vi "Edit Line.vi"(8 "error in":errorcluster, 10 "Line Name":string, 11 "References":T1) -> (0 "error out":errorcluster, 2 "change?":bool)   [LabVIEW 2014, in "Missing Plugin editor node.lvclass"]
doc: "This VI edits the properties of a line. It will unlink channels and tags and create new links to channels and tags."
uses:
  Missing Plugin editor node.lvclass
  <vilib>/NI/DCAF/Tag Editor Core/Table API/Table Manager/object ref.ctl
  <vilib>/NI/DCAF/Tag Editor Core/Configuration Editor/Classes/Engine Parent/Engine Parent Editor Node.lvclass
  <vilib>/NI/DCAF/Tag Editor Core/Configuration Editor/Classes/Module editor node/module editor node.lvclass
  module/configuration/Missing Plugin configuration.lvclass
  module/configuration/Missing Plugin configuration.lvclass/Missing Plugin configuration.ctl
  <vilib>/NI/Configuration Framework/serializable configuration/NISE_CEF_serializable configuration.lvclass/NISE_CEF_serializable configuration.ctl
  <vilib>/Utility/LVClass/Get LV Class Name.vi
  <vilib>/NI/Configuration Framework/error generator/NISE_error generator.vi
  <vilib>/NI/Tag Bus Module Framework/channel/TBM channel.lvclass
  <vilib>/NI/Configuration Framework/serializable configuration/NISE_CEF_serializable configuration.lvclass
  <vilib>/NI/DCAF/Tag Editor Core/Table API/Table Manager/Table Manager.lvclass
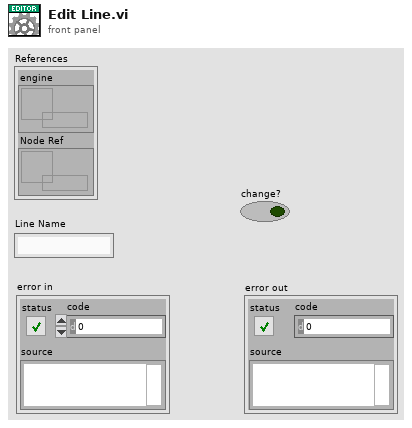
[diagram p1: front panel]
types:
  T1 = typedef "Table Manager.lvlib/Table Manager.lvclass/object ref.ctl" = cluster{"engine":refnum<data-value>, "Node Ref":refnum<data-value>}
  T2 = typedef "Missing Plugin configuration.lvclass/Line.ctl" = cluster{"channel":refnum<class "TBM channel.lvclass">}
  T3 = typedef "Missing Plugin editor node.lvclass/Mappings.ctl" = cluster{"Line":T2, "Maps":T4[]}
  T4 = typedef "Missing Plugin editor node.lvclass/Map.ctl" = cluster{"channel":refnum<class "TBM channel.lvclass">, "tag name":string}
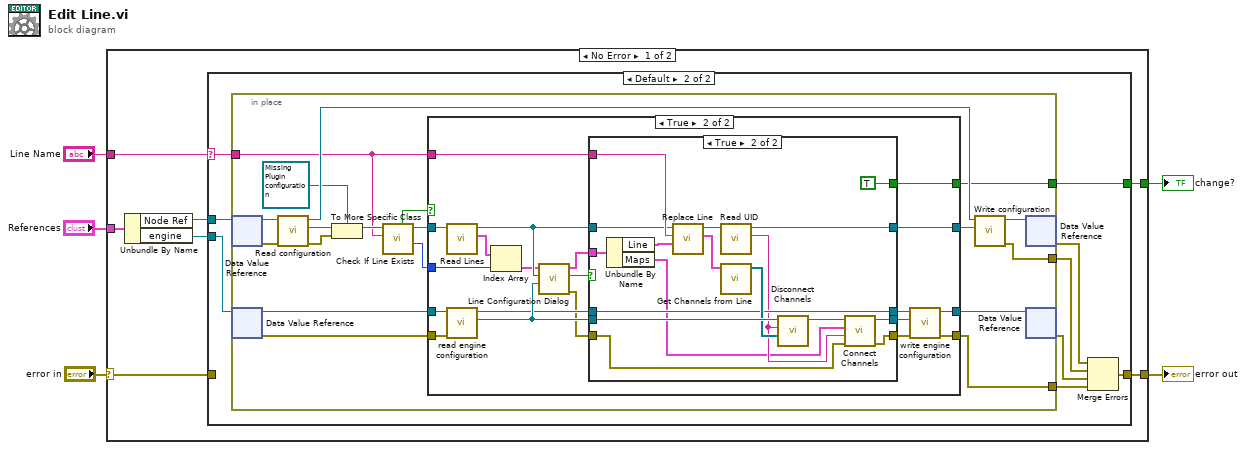
[diagram p0: block diagram]
diagram:
  n1 = case shown="No Error" "error in" {
    selector: "error in" -> [w6 w86]
    tunnel: "References" -> [w10 _]
    tunnel: "Line Name" -> [w7 _]
    tunnel: [w9 w86] -> w2
    tunnel: [w8 _] -> w1
    frame No Error {
      n2 = Unbundle By Name(w10) -> ("Node Ref"=w12:refnum<data-value>, "engine"=w11:refnum<data-value>)
      n3 = case shown="Default" w7 {
        selector: w7 -> [_ w16]
        tunnel: w12 -> [_ w22]
        tunnel: w11 -> [_ w21]
        tunnel: [w13 w18] -> w9
        tunnel: [_ w17] -> w8
        tunnel: w6 -> [w13 _]
        frame " " {
        }
        frame Default {
          n4 = in-place {
            in-place-border: [w29] -> w20
            in-place-border: [w23] -> w19
            in-place-border: [w28] -> w17
            in-place-border: w16 -> [w33]
            n5 = in-place-dvr #1(w22) -> (w40:refnum<class "module editor node.lvclass">, w34:errorcluster)
            n6 = in-place-dvr #2(w21) -> (w26:refnum<class "Engine Parent Editor Node.lvclass">, w25:errorcluster)
            n7 = call-dynamic "Read configuration.vi"("error in"=w34, "NISE_CEF_serializable node in"=w40) -> ("error out"=w37:errorcluster, "configuration"=w38:refnum<class "NISE_CEF_serializable configuration.lvclass">, "NISE_CEF_serializable node out"=w39:refnum<class "module editor node.lvclass">)  [unwired: 7 in]
            n8 = To More Specific Class(target class=refnum<class "Missing Plugin configuration.lvclass"> refnum ("tag bus configurable plugin module configuration"), reference=w38, error in=w37) -> (specific class reference=w35:refnum<class "Missing Plugin configuration.lvclass">)  [unwired: 1 out]
            n9 = call-dynamic "Check If Line Exists.vi"("Name to Locate"=w33, "Missing Plugin configuration in"=w35) -> ("Index"=w30:i32, "Missing Plugin configuration out"=w31:refnum<class "Missing Plugin configuration.lvclass">, "Found?"=w27:bool)  [unwired: 5 in, 2 out]
            n10 = case shown="True" w27 {
              tunnel: w31 -> [w44 w63]
              tunnel: w33 -> [_ w64]
              tunnel: [w44 w57] -> w32
              tunnel: w30 -> [_ w60]
              tunnel: [_ w55] -> w28
              tunnel: w26 -> [w43 w54]
              tunnel: w25 -> [w42 w53]
              tunnel: [w43 w51] -> w24
              tunnel: [w42 w50] -> w23
              frame False {
              }
              frame True {
                n11 = call "Read Lines.vi"("Missing Plugin configuration in"=w63) -> ("Lines"=w61:T2[], "Missing Plugin configuration out"=w62:refnum<class "Missing Plugin configuration.lvclass">)  [unwired: 8 in, 1 out]
                n12 = call <vilib>:"read engine configuration.vi"("error in"=w53, "Engine Parent Editor Node in"=w54) -> ("engine configuration"=w52:refnum<class "engine configuration.lvclass">, "Engine Parent Editor Node out"=w48:refnum<class "Engine Parent Editor Node.lvclass">)  [unwired: 7 in, 1 out]
                n13 = Index Array(array=w61, index=w60) -> (element=w59:T2)
                n14 = call "Line Configuration Dialog.vi"("engine configuration in"=w52, "tag bus configurable plugin module configuration"=w62, "Line"=w59) -> ("error out"=w45:errorcluster, "changed"=w56:bool, "Mappings out"=w58:T3)  [unwired: 5 in, 1 out]
                n15 = case shown="True" w56 {
                  tunnel: w64 -> [_ w85]
                  tunnel: w52 -> [w67 w84]
                  tunnel: w62 -> [w68 w80]
                  tunnel: w58 -> [_ w79]
                  tunnel: [w68 w77] -> w57
                  tunnel: [_ TRUE ("change?")] -> w55
                  tunnel: [w67 w74] -> w47
                  tunnel: [w66 w73] -> w49
                  tunnel: w48 -> [w66 w73]
                  tunnel: [w65 w70] -> w46
                  tunnel: w45 -> [w65 w71]
                  frame False {
                  }
                  frame True {
                    n16 = Unbundle By Name(w79) -> ("Line"=w78:T2, "Maps"=w69:T4[])
                    n17 = call "Replace Line.vi"("New Line"=w78, "Line Name"=w85, "Missing Plugin configuration in"=w80) -> ("Old Line"=w82:T2, "Missing Plugin configuration out"=w83:refnum<class "Missing Plugin configuration.lvclass">)  [unwired: 6 in, 1 out]
                    n18 = call <vilib>:"Read UID.vi"("configuration in"=w83) -> ("instance id"=w72:string, "configuration out"=w77:refnum<class "Missing Plugin configuration.lvclass">)  [unwired: 8 in, 1 out]
                    n19 = call "Get Channels from Line.vi"("Line"=w82) -> ("Channels"=w81:refnum<class "TBM channel.lvclass">[])  [unwired: 10 in]
                    n20 = call "Disconnect Channels.vi"("Deleted Channels"=w81, "instance id"=w72, "Engine Configuration in"=w84) -> ("Engine Configuration out"=w76:refnum<class "engine configuration.lvclass">)  [unwired: 7 in, 1 out]
                    n21 = call "Connect Channels.vi"("error in (no error)"=w71, "instance id"=w72, "Maps"=w69, "Engine Configuration in"=w76) -> ("error out"=w70:errorcluster, "Engine Configuration out"=w74:refnum<class "engine configuration.lvclass">)  [unwired: 6 in]
                  }
                }
                n22 = call <vilib>:"write engine configuration.vi"("error in"=w46, "engine configuration"=w47, "Engine Parent Editor Node in"=w49) -> ("error out"=w50:errorcluster, "Engine Parent Editor Node out"=w51:refnum<class "Engine Parent Editor Node.lvclass">)  [unwired: 7 in]
              }
            }
            n23 = call-dynamic "Write configuration.vi"("configuration"=w32, "NISE_CEF_serializable node in"=w39) -> ("error out"=w29:errorcluster, "NISE_CEF_serializable node out"=w41:refnum<class "module editor node.lvclass">)  [unwired: 8 in]
            n24 = in-place-dvr #1(w41) -> (w14:errorcluster)  [unwired: 1 out]
            n25 = in-place-dvr #2(w24) -> (w15:errorcluster)  [unwired: 1 out]
          }
          n26 = Merge Errors(w14, w20, w15, w19) -> (w18:errorcluster)
        }
      }
    }
    frame Error {
    }
  }
  "change?" <- w1
  "error out" <- w2
